vi "Font - Heading 3 Font Tests.vi"(8 "error in (no error)":errorcluster) -> (0 "error out":errorcluster)   [LabVIEW 2020]
uses:
  src/Font/Font/Underline--ring.ctl
  src/Font/Font/Alignment--ring.ctl
  src/Font/Heading 3/Heading 3.lvclass
  D:/Benjamin/Documents/Perso/Code/WC/LabVIEW_NPOI/src/Font/Font/Font.lvclass
  src/Font/Font/Get Color (Hex).vi
  <vilib>/addons/_JKI Toolkits/Caraya/classes/Assert/Assert Equal Value and Type_Variant.vi
  <vilib>/addons/_JKI Toolkits/Caraya/classes/Assert/Assert False.vi
  <vilib>/addons/_JKI Toolkits/Caraya/classes/Assert/Assert Equal Value_Variant.vi
  <vilib>/addons/_JKI Toolkits/Caraya/classes/Test/Test.lvclass
  <vilib>/addons/_JKI Toolkits/Caraya/classes/Assert/Assert.lvclass
  src/Font/Font/Font.lvclass
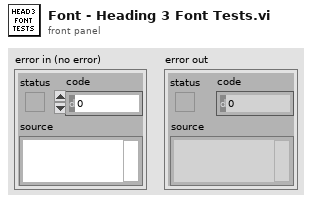
[diagram p1: front panel]
types:
  T1 = typedef "Fonts.lvlib/Font.lvclass/Alignment--ring.ctl" = i32
  T2 = typedef "Fonts.lvlib/Font.lvclass/Underline--ring.ctl" = i32
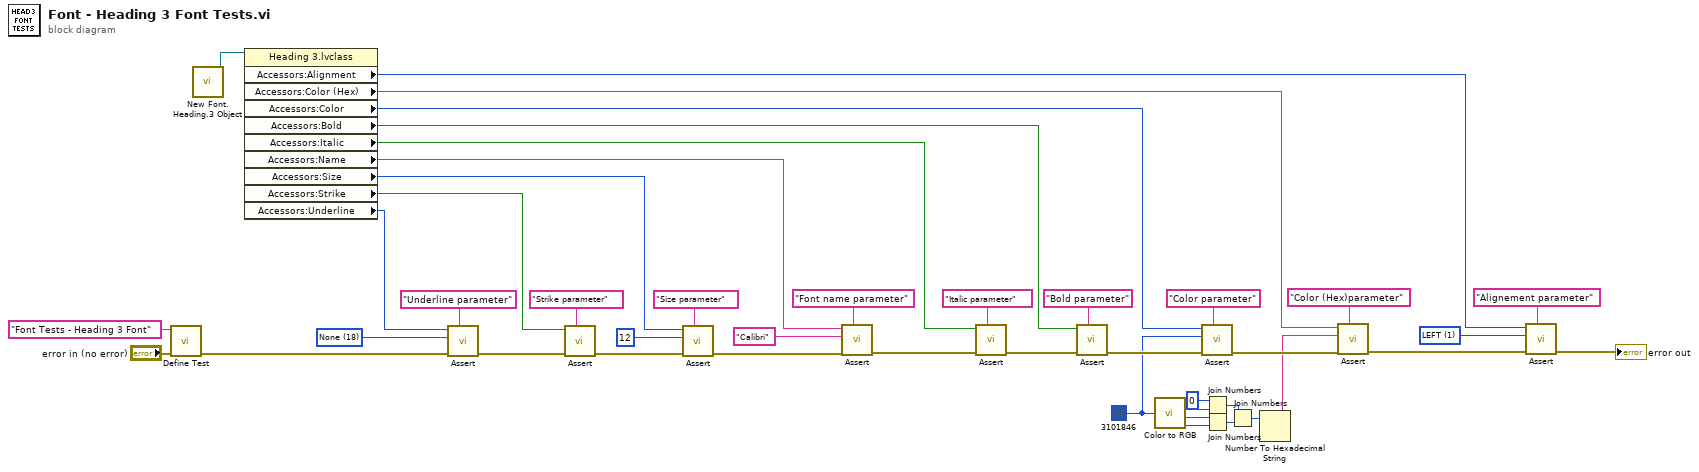
[diagram p0: block diagram]
diagram:
  w4 = T1 1 items=["LEFT"=1, "CENTER"=2, "RIGHT"=3, "BOTH"=4, "MEDIUM_KASHIDA"=5, "DISTRIBUTE"=6, "NUM_TAB"=7, "HIGH_KASHIDA"=8, "LOW_KASHIDA"=9, "THAI_DISTRIBUTE"=10] ("Style:Alignment")
  w10 = u32 3101846 ("Color")
  w32 = T2 18 items=["Single"=1, "Words"=2, "Double"=3, "Thick"=4, "Dotted"=5, "DottedHeavy"=6, "Dash"=7, "DashedHeavy"=8, "DashLong"=9, "DashLongHeavy"=10, "DotDash"=11, "DashDotHeavy"=12, "DotDotDash"=13, "DashDotDotHeavy"=14, "Wave"=15, "WavyHeavy"=16, "WavyDouble"=17, "None"=18] ("Style:Underline")
  n1 = call <vilib>:"Define Test.vi"("error in (no error)"="error in (no error)", "Label (VI Title)"="Font Tests - Heading 3 Font") -> ("error out"=w44:errorcluster)  [unwired: 9 in]
  n2 = call "New Font.Heading.3 Object.vi"() -> ("Heading 3 out"=w34:refnum<class "Heading 3.lvclass">)  [unwired: 10 in, 1 out]
  n3 = property class="Heading 3.lvclass"(reference=w34) -> ("Accessors:Alignment"=w1:T1, "Accessors:Color (Hex)"=w7:string, "Accessors:Color"=w11:u32, "Accessors:Bold"=w21:bool, "Accessors:Italic"=w25:bool, "Accessors:Name"=w28:string, "Accessors:Size"=w30:i32, "Accessors:Strike"=w31:bool, "Accessors:Underline"=w33:T2)  [unwired: 1 in, 2 out]
  n4 = call-poly <vilib>:"Assert.vi"("Label"="Underline parameter", "error in (no error)"=w44, "Y"=w32, "X"=w33) -> ("error out"=w42:errorcluster)  [unwired: 7 in]
  n5 = call-poly <vilib>:"Assert.vi"("Label"="Strike parameter", "error in (no error)"=w42, "False?"=w31) -> ("error out"=w37:errorcluster)  [unwired: 8 in]
  n6 = call-poly <vilib>:"Assert.vi"("Label"="Size parameter", "error in (no error)"=w37, "Y"=12 ("Style:Size"), "X"=w30) -> ("error out"=w36:errorcluster)  [unwired: 7 in]
  n7 = call-poly <vilib>:"Assert.vi"("Label"="Font name parameter", "error in (no error)"=w36, "Y"="Calibri" ("Label"), "X"=w28) -> ("error out"=w24:errorcluster)  [unwired: 7 in]
  n8 = call-poly <vilib>:"Assert.vi"("Label"="Italic parameter", "error in (no error)"=w24, "False?"=w25) -> ("error out"=w22:errorcluster)  [unwired: 8 in]
  n9 = call-poly <vilib>:"Assert.vi"("Label"="Bold parameter", "error in (no error)"=w22, "False?"=w21) -> ("error out"=w12:errorcluster)  [unwired: 8 in]
  n10 = call <vilib>:"Color to RGB.vi"("Color"=w10) -> ("R"=w20:u8, "G"=w19:u8, "B"=w18:u8)  [unwired: 1 out]
  n11 = call-poly <vilib>:"Assert.vi"("Label"="Color parameter", "error in (no error)"=w12, "Y"=w10, "X"=w11) -> ("error out"=w8:errorcluster)  [unwired: 7 in]
  n12 = Join Numbers(hi=u8 0, lo=w20) -> ((hi.lo)=w16:u16)
  n13 = Join Numbers(hi=w19, lo=w18) -> ((hi.lo)=w15:u16)
  n14 = Join Numbers(hi=w16, lo=w15) -> ((hi.lo)=w14:u32)
  n15 = Number To Hexadecimal String(2:w14) -> (0:w6:string)  [unwired: 1 in]
  n16 = call-poly <vilib>:"Assert.vi"("Label"="Color (Hex)parameter", "error in (no error)"=w8, "Y"=w6, "X"=w7) -> ("error out"=w3:errorcluster)  [unwired: 7 in]
  n17 = call-poly <vilib>:"Assert.vi"("Label"="Alignement parameter", "error in (no error)"=w3, "Y"=w4, "X"=w1) -> ("error out"=→"error out":errorcluster)  [unwired: 7 in]
